vi "FFT.vi"   [LabVIEW 2016, in "xy_utilities.lvlib"]
uses:
  xy_utilities.lvlib
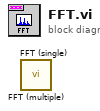
[diagram p0: block diagram]
diagram:
  n1 = call "FFT (multiple).vi"() -> ()  [unwired: 8 in, 4 out]
  n2 = call "FFT (single).vi"() -> ()  [unwired: 8 in, 4 out]
